vi "load_boat_icons.vi"() -> (3 "Boat Overlay References Out":T2)   [LabVIEW 2013]
doc: "Loads the boat icon for use on the map. Also, replaces all the black pixels with transparent pixels.\n\n4/5/2014\nMac-I Crowell"
uses:
  TypeDef/boat_overlay_references.ctl
  <vilib>/vision/Image Controls.llb/IMAQ Image.ctl
panel:
  out "Main Image":T1(plugin-control)
  out "Jib Image":T1(plugin-control)
  out "Rudder Image":T1(plugin-control)
  out "Boat Image":T1(plugin-control)
  out "appended boat icon path":path
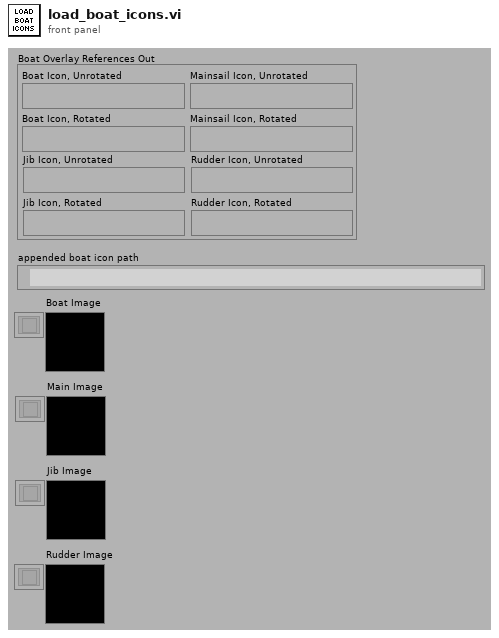
[diagram p1: front panel]
types:
  T1 = typedef "IMAQ Image.ctl" = refnum<image>
  T2 = typedef "boat_overlay_references.ctl" = cluster{"Boat Icon, Unrotated":T1, "Boat Icon, Rotated":T1, "Mainsail Icon, Unrotated":T1, "Mainsail Icon, Rotated":T1, "Jib Icon, Rotated":T1, "Jib Icon, Unrotated":T1, "Rudder Icon, Rotated":T1, "Rudder Icon, Unrotated":T1}
  T3 = typedef "Image Type" = u32
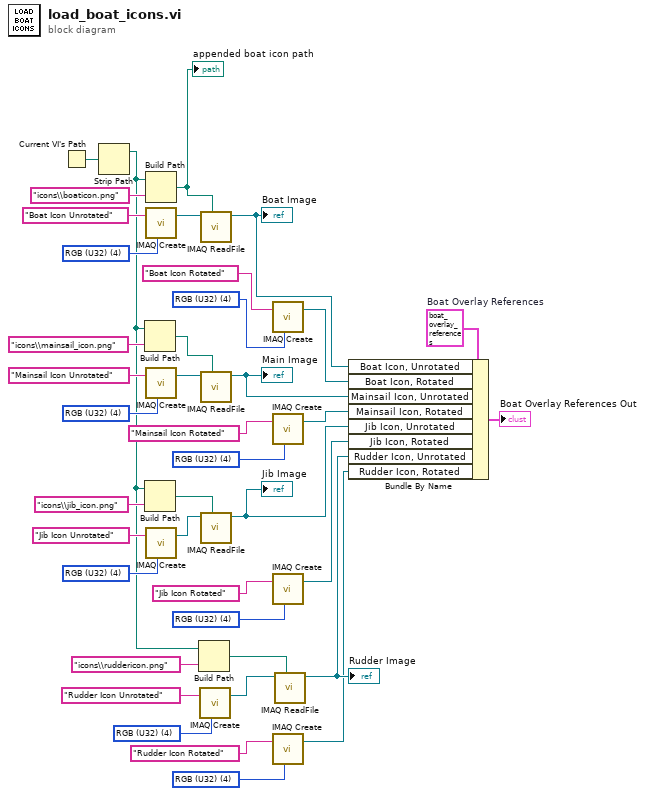
[diagram p0: block diagram]
diagram:
  w8 = T3 4 items=["Grayscale (U8)", "Grayscale (I16)", "Grayscale (SGL)", "Complex (CSG)", "RGB (U32)", "HSL (U32)", "RGB (U64)", "Grayscale (U16)"] ("Image Type")
  w9 = T3 4 items=["Grayscale (U8)", "Grayscale (I16)", "Grayscale (SGL)", "Complex (CSG)", "RGB (U32)", "HSL (U32)", "RGB (U64)", "Grayscale (U16)"] ("Image Type")
  w19 = T3 4 items=["Grayscale (U8)", "Grayscale (I16)", "Grayscale (SGL)", "Complex (CSG)", "RGB (U32)", "HSL (U32)", "RGB (U64)", "Grayscale (U16)"] ("Image Type")
  w18 = T3 4 items=["Grayscale (U8)", "Grayscale (I16)", "Grayscale (SGL)", "Complex (CSG)", "RGB (U32)", "HSL (U32)", "RGB (U64)", "Grayscale (U16)"] ("Image Type")
  w21 = T2 {"Boat Icon, Unrotated"=refnum, "Boat Icon, Rotated"=refnum, "Mainsail Icon, Unrotated"=refnum, "Mainsail Icon, Rotated"=refnum, "Jib Icon, Rotated"=refnum, "Jib Icon, Unrotated"=refnum, "Rudder Icon, Rotated"=refnum, "Rudder Icon, Unrotated"=refnum}  # Boat Overlay References
  w27 = T3 4 items=["Grayscale (U8)", "Grayscale (I16)", "Grayscale (SGL)", "Complex (CSG)", "RGB (U32)", "HSL (U32)", "RGB (U64)", "Grayscale (U16)"] ("Image Type")
  w28 = T3 4 items=["Grayscale (U8)", "Grayscale (I16)", "Grayscale (SGL)", "Complex (CSG)", "RGB (U32)", "HSL (U32)", "RGB (U64)", "Grayscale (U16)"] ("Image Type")
  w33 = T3 4 items=["Grayscale (U8)", "Grayscale (I16)", "Grayscale (SGL)", "Complex (CSG)", "RGB (U32)", "HSL (U32)", "RGB (U64)", "Grayscale (U16)"] ("Image Type")
  w40 = T3 4 items=["Grayscale (U8)", "Grayscale (I16)", "Grayscale (SGL)", "Complex (CSG)", "RGB (U32)", "HSL (U32)", "RGB (U64)", "Grayscale (U16)"] ("Image Type")
  n1 = Current VI's Path() -> (path=w37:path)
  n2 = Strip Path(path=w37) -> (stripped path=w5:path)  [unwired: 1 out]
  n3 = Build Path(base path=w5, name or relative path="icons\\mainsail_icon.png") -> (appended path=w32:path)
  n4 = Build Path(base path=w5, name or relative path="icons\\jib_icon.png") -> (appended path=w14:path)
  n5 = Build Path(base path=w5, name or relative path="icons\\boaticon.png") -> (appended path=w35:path)
  "appended boat icon path" <- w35
  n6 = call "IMAQ Create"("Image Name"="Boat Icon Unrotated", "Image Type"=w40) -> ("New Image"=w38:T1)  [unwired: 2 in, 2 out]
  n7 = call "IMAQ Create"("Image Name"="Mainsail Icon Unrotated", "Image Type"=w28) -> ("New Image"=w30:T1)  [unwired: 2 in, 2 out]
  n8 = call "IMAQ Create"("Image Name"="Jib Icon Unrotated", "Image Type"=w18) -> ("New Image"=w16:T1)  [unwired: 2 in, 2 out]
  n9 = Build Path(base path=w5, name or relative path="icons\\ruddericon.png") -> (appended path=w13:path)
  n10 = call "IMAQ Create"("Image Name"="Rudder Icon Unrotated", "Image Type"=w9) -> ("New Image"=w11:T1)  [unwired: 2 in, 2 out]
  n11 = call "IMAQ ReadFile"("File Path"=w35, "Image"=w38) -> ("Image Out"=w23:T1)  [unwired: 3 in, 6 out]
  "Boat Image" <- w23
  n12 = call "IMAQ ReadFile"("File Path"=w32, "Image"=w30) -> ("Image Out"=w1:T1)  [unwired: 3 in, 6 out]
  "Main Image" <- w1
  n13 = call "IMAQ ReadFile"("File Path"=w14, "Image"=w16) -> ("Image Out"=w2:T1)  [unwired: 3 in, 6 out]
  "Jib Image" <- w2
  n14 = call "IMAQ Create"("Image Name"="Boat Icon Rotated", "Image Type"=w33) -> ("New Image"=w24:T1)  [unwired: 2 in, 2 out]
  n15 = call "IMAQ Create"("Image Name"="Mainsail Icon Rotated", "Image Type"=w27) -> ("New Image"=w25:T1)  [unwired: 2 in, 2 out]
  n16 = call "IMAQ Create"("Image Name"="Jib Icon Rotated", "Image Type"=w19) -> ("New Image"=w6:T1)  [unwired: 2 in, 2 out]
  n17 = call "IMAQ Create"("Image Name"="Rudder Icon Rotated", "Image Type"=w8) -> ("New Image"=w3:T1)  [unwired: 2 in, 2 out]
  n18 = call "IMAQ ReadFile"("File Path"=w13, "Image"=w11) -> ("Image Out"=w4:T1)  [unwired: 3 in, 6 out]
  "Rudder Image" <- w4
  n19 = Bundle By Name(cluster=w21, "Boat Icon, Unrotated"=w23, "Boat Icon, Rotated"=w24, "Mainsail Icon, Unrotated"=w1, "Mainsail Icon, Rotated"=w25, "Jib Icon, Unrotated"=w2, "Jib Icon, Rotated"=w6, "Rudder Icon, Unrotated"=w4, "Rudder Icon, Rotated"=w3) -> (→"Boat Overlay References Out":T2)
